vi "Kalman Filter.vi"(6 "Observations2\naccelerometer angle":dbl format="%#_13g", 7 "Observations1\nGyro":dbl format="%#_13g", 9 "F  Matrix":T1, 10 "H Matrix":T1, 11 "Steady State Kalman Predictor Gain matrixx":T1) -> (3 "State Predicted Estimate X^(k+1/k)":dbl[](array[numeric]))   [LabVIEW 2016]
uses:
  <vilib>/Analysis/Matrix/Datatypes/RealMatrix.ctl
  <vilib>/Analysis/Matrix/NI_Matrix.lvlib
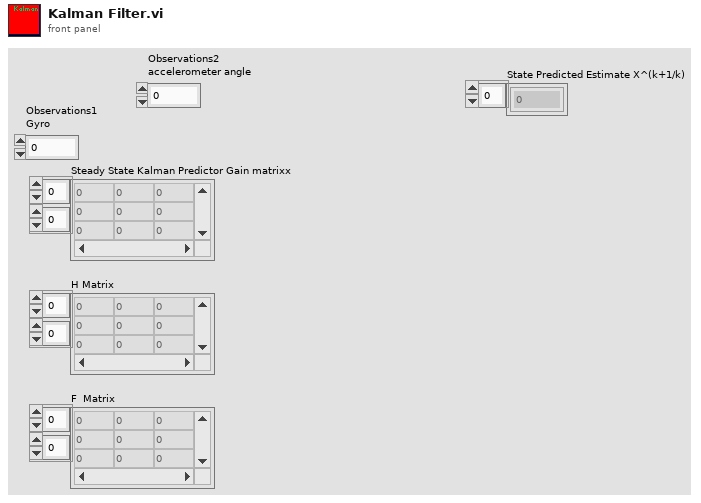
[diagram p1: front panel]
types:
  T1 = typedef "NI_Matrix.lvlib/RealMatrix.ctl" = dbl[][]
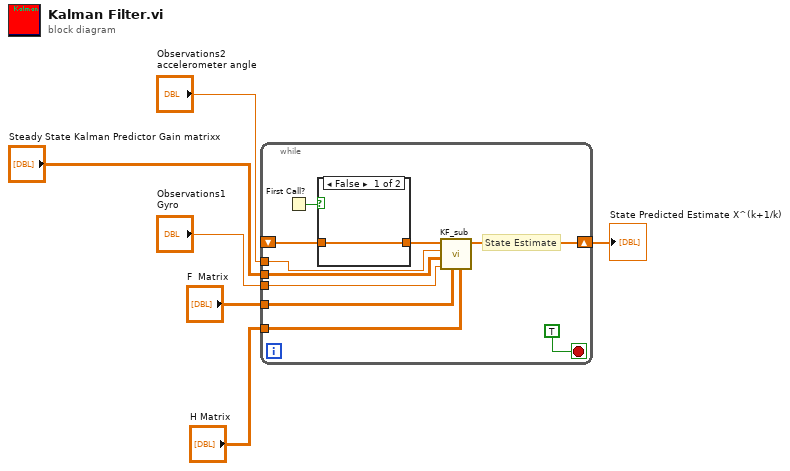
[diagram p0: block diagram]
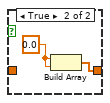
[diagram p2: hidden frame]
diagram:
  n1 = while {
    tunnel: "Steady State Kalman Predictor Gain matrixx" -> [w16]
    tunnel: "F  Matrix" -> [w15]
    tunnel: "H Matrix" -> [w14]
    shift-right: [w13] -> w3
    shift-left: _ -> [w10]
    tunnel: "Observations2\naccelerometer angle" -> [w8]
    tunnel: "Observations1\nGyro" -> [w7]
    stop <- TRUE stop-if-true
    # "State Estimate"
    n2 = First Call?() -> (First Call?: T/F=w11:bool)
    n3 = case shown="False" w11 {
      tunnel: w10 -> [w17 _]
      tunnel: [w17 w18] -> w9
      frame False {
      }
      frame True {
        w19 = 0.0 ("element")
        n4 = Build Array(w19, w19) -> (w18:dbl[])
      }
    }
    n5 = call "KF_sub.vi"("H Matrix"=w14, "F  Matrix"=w15, "Observations 1 Gyro Velocity"=w7, "Steady State Kalman Predictor Gain matrix"=w16, "Observations 2 Accelerometer ANGLE in degrees"=w8, "X from register"=w9) -> ("X^ to register"=w13:dbl[])  [unwired: 5 in]
  }
  "State Predicted Estimate X^(k+1/k)" <- w3
